vi "Text Markup.vi"() -> ()   [LabVIEW 2013]
uses:
  <vilib>/Heliosphere Research LLC/Advanced Plotting Toolkit/api_annotations/TextProperties.ctl
  <vilib>/Heliosphere Research LLC/Advanced Plotting Toolkit/properties/Text.ctl
  <vilib>/Heliosphere Research LLC/Advanced Plotting Toolkit/typedefs/PlotColor.ctl
  <vilib>/Heliosphere Research LLC/Advanced Plotting Toolkit/properties/Text_FontSize.ctl
  <vilib>/Heliosphere Research LLC/Advanced Plotting Toolkit/properties/Text_FontStyle.ctl
  <vilib>/Heliosphere Research LLC/Advanced Plotting Toolkit/properties/Display.ctl
  <vilib>/Heliosphere Research LLC/Advanced Plotting Toolkit/Advanced Plotting Toolkit.lvlib
panel:
  in  "Text":string="$g(m,x) = \\frac{2\\pi}{\\sqrt{m}} \\sum_{i=0}^{\\infty} \\sin{x_i}$"
  out "Text Example":picture
  # "Inline Text Markup"
  # "This example demonstrates the use of math markup.  Math\nmarkup can be used anywhere text is displayed on a plot.  This\nexample uses Text.vi, but you can also use inline markup on\naxis labels, plot titles, legend names, etc.\n\nThe mini-language used for markup is LaTeX.  Enter \"math\nmode\" by surrounding an expression in the string with\ndollar signs ($).  Everything between the dollar signs will be\nprocessed by the markup engine.\n\nFor an introduction to using this feature, and a list of\nsupported markup constructs, consult the user manual section\n\"Using Inline Text Markup\"."
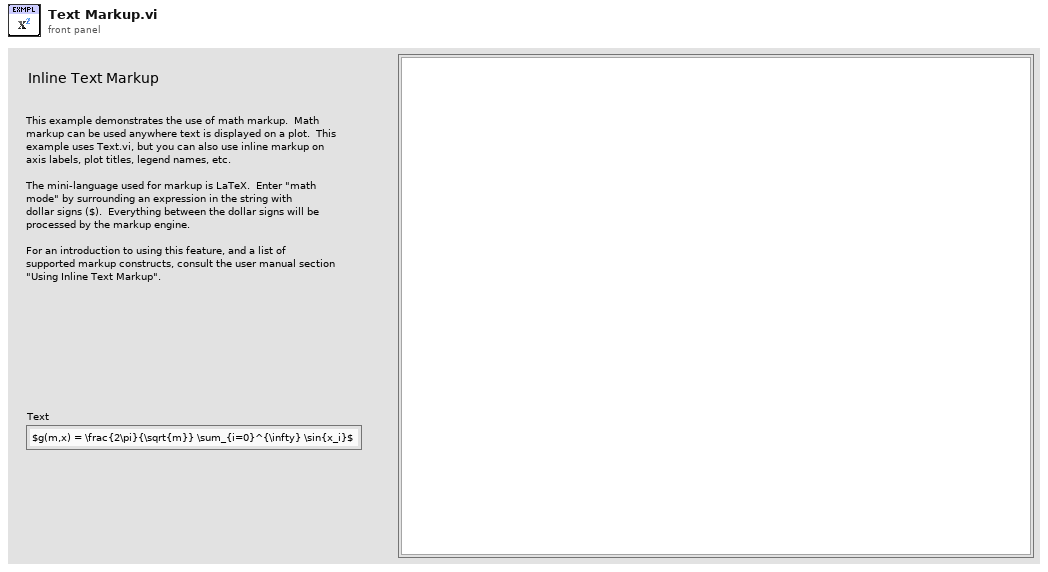
[diagram p1: front panel]
types:
  T1 = typedef "Advanced Plotting Toolkit.lvlib/TextProperties.ctl" = cluster{"Text":T2, "Display":T6}
  T2 = typedef "Advanced Plotting Toolkit.lvlib/Text.ctl" = cluster{"Color":T3, "Background Color":T3, "Font Size (points)":T4, "Font Style":T5, "Rotation Angle":dbl}
  T3 = typedef "Advanced Plotting Toolkit.lvlib/PlotColor.ctl" = u32
  T4 = typedef "Advanced Plotting Toolkit.lvlib/Text_FontSize.ctl" = i32
  T5 = typedef "Advanced Plotting Toolkit.lvlib/Text_FontStyle.ctl" = enum16{"Automatic", "Normal", "Italic", "Bold"}
  T6 = typedef "Advanced Plotting Toolkit.lvlib/Display.ctl" = cluster{"Alpha":dbl, "Z Order":dbl}
  T7 = typedef "Advanced Plotting Toolkit.lvlib/PlotID.ctl" = i32
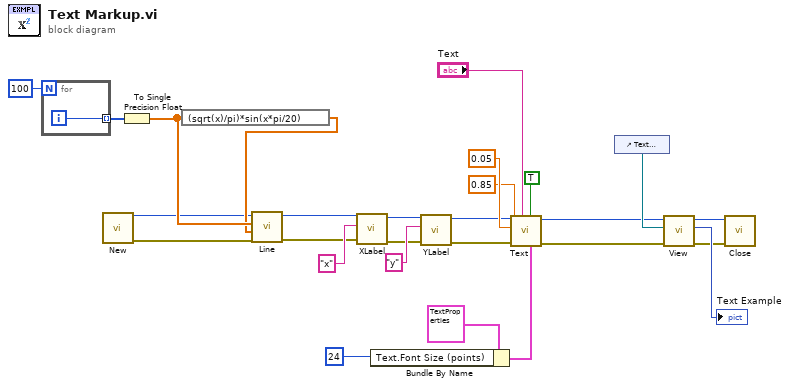
[diagram p0: block diagram]
diagram:
  n1 = for {
    N: 100 -> [_]
    tunnel: [w28] -> w23 mode=indexing
    i -> [w28]
  }
  n2 = call <vilib>:"New.vi"() -> ("error out"=w7:errorcluster, "Plot ID"=w20:T7)  [unwired: 10 in]
  n3 = To Single Precision Float(number=w23) -> (single precision float=w22:sgl[])
  n4 = expression code="(sqrt(x)/pi)*sin(x*pi/20)"(w22) -> (w21:sgl[])
  n5 = call <vilib>:"Line.vi"("error in (no error)"=w7, "Y Data"=w21, "X Data"=w22, "Plot ID"=w20) -> ("error out"=w6:errorcluster, "Plot ID out"=w19:T7)  [unwired: 6 in]
  n6 = call <vilib>:"XLabel.vi"("error in (no error)"=w6, "Label"="x", "Plot ID"=w19) -> ("error out"=w5:errorcluster, "Plot ID out"=w17:T7)  [unwired: 7 in]
  n7 = Bundle By Name(cluster=T1 {"Text"={"Color"=2147483647, "Background Color"=2147483647, "Font Size (points)"=0, "Font Style"=enum."Automatic", "Rotation Angle"=nan}, "Display"={"Alpha"=nan, "Z Order"=nan}} ("Text Properties"), "Text.Font Size (points)"=24) -> (w8:T1)
  n8 = call <vilib>:"YLabel.vi"("error in (no error)"=w5, "Label"="y", "Plot ID"=w17) -> ("error out"=w4:errorcluster, "Plot ID out"=w12:T7)  [unwired: 7 in]
  n9 = call <vilib>:"Text.vi"("Properties"=w8, "Relative Coordinates"=TRUE, "Text"="Text", "error in (no error)"=w4, "Y Position"=0.85, "X Position"=0.05, "Plot ID"=w12) -> ("error out"=w3:errorcluster, "Plot ID Out"=w11:T7)  [unwired: 3 in]
  n10 = control-ref of="Text Example"() -> (w26:refnum<vi>)
  n11 = call <vilib>:"View.vi"("error in (no error)"=w3, "Ref for Sizing"=w26, "Plot ID"=w11) -> ("error out"=w1:errorcluster, "Picture"=→"Text Example":picture, "Plot ID Out"=w25:T7)  [unwired: 6 in]
  n12 = call <vilib>:"Close.vi"("error in (no error)"=w1, "Plot ID"=w25) -> ()  [unwired: 9 in, 1 out]
